vi "gfitsio-write-image-subset-i16-3d.vi"(6 "fpixel (1,1,1)":cluster{"X":i32, "Y":i32, "Z":i32}={"X"=1, "Y"=1, "Z"=1}, 8 "error in (no error)":errorcluster, 9 "data":i16[][][](array[numeric]), 11 "gfits refnum":T1) -> (0 "error out":errorcluster, 3 "dup gfits refnum":T1)   [LabVIEW 2011, in "gfitsio.lvlib"]
doc: "Write a rectangular subimage (or the whole image) to the FITS data array. <B>fpixel</B> gives the coordinates of the lower left corner of the subset to which you want to write. The default is the lower left corner of the image."
uses:
  gfitsio.lvlib
  gfitsio-refnum.ctl
  cfitsio-hdutypes.ctl
  gfitsio.dll
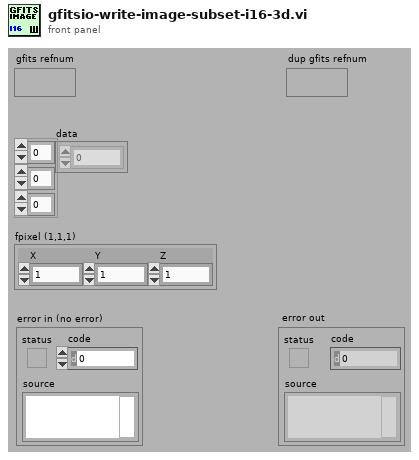
[diagram p1: front panel]
types:
  T1 = typedef "gfitsio.lvlib/gfitsio-refnum.ctl" = refnum<k1>
  T2 = typedef "gfitsio.lvlib/cfitsio-hdutypes.ctl" = i32
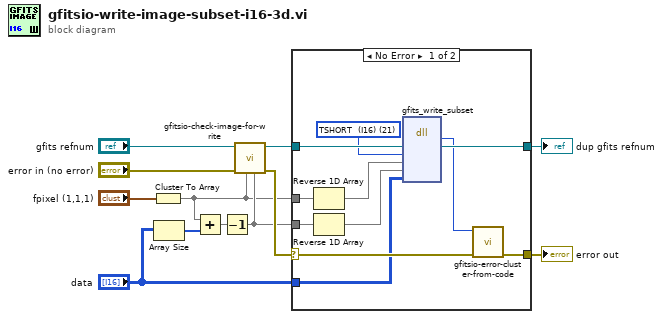
[diagram p0: block diagram]
diagram:
  n1 = Cluster To Array(cluster="fpixel (1,1,1)") -> (array=w1:i32[])
  n2 = Array Size(array="data") -> (size(s)=w2:i32[])
  n3 = Add(x=w1, y=w2) -> (x+y=w4:i32[])
  n4 = Decrement(x=w4) -> (x-1=w3:i32[])
  n5 = call "gfitsio-check-image-for-write.vi"("lpixel"=w3, "fpixel"=w1, "error in (no error)"="error in (no error)", "gfits refnum"="gfits refnum") -> ("error out"=w7:errorcluster, "dup gfits refnum"=w9:T1)  [unwired: 6 in]
  n6 = case shown="No Error" w7 {
    selector: w7 -> [w23 w25]
    tunnel: [w22 w25] -> w12
    tunnel: [w20 w24] -> w11
    tunnel: w9 -> [w21 w24]
    tunnel: "data" -> [w17 _]
    tunnel: w1 -> [w13 _]
    tunnel: w3 -> [w16 _]
    frame No Error {
      w18 = T2 21 items=["TBIT"=1, "TBYTE  (U8)"=11, "TSBYTE  (I8)"=12, "TLOGICAL"=14, "TSTRING"=16, "TUSHORT  (U16)"=20, "TSHORT  (I16)"=21, "TUINT"=31, "TULONG  (U32)"=40, "TLONG  (I32)"=41, "TFLOAT  (SGL)"=42, "TLONGLONG  (I64)"=81, "TDOUBLE"=82, "TCOMPLEX  (CSG)"=83, "TDOUBLECOMPLEX  (CDB)"=163] ("cfitsio datatype")
      n7 = Reverse 1D Array(array=w13) -> (reversed array=w14:i32[])
      n8 = Reverse 1D Array(array=w16) -> (reversed array=w15:i32[])
      n9 = dll-call lib="C:/BonOMM/BonOMM-2012/SubVIs/gfitsio/gfitsio.dll" fn="gfits_write_subset"("dup gfits refnum"=w21, "datatype"=w18, "fpixel"=w14, "lpixel"=w15, "array"=w17) -> (w19:i32, "dup gfits refnum"=w20:T1)  [unwired: 7 in, 2 out]
      n10 = call "gfitsio-error-cluster-from-code.vi"("error in (no error)"=w23, "error code"=w19) -> ("error out"=w22:errorcluster)  [unwired: 9 in]
    }
    frame Error {
    }
  }
  "error out" <- w12
  "dup gfits refnum" <- w11
